vi "Pose_Estimation.vi"() -> ()   [LabVIEW 2019]
uses:
  Hardware/Drive/Drive_Hardware_Globals.vi
  <vilib>/Rock Robotics/WPI/ThirdParty/Phoenix-LabVIEW/Motor Controller/Get/CTRE_Phoenix_MotorController_GetSelectedSensorData.vi
  Globals/Sensor_Values.vi
panel:
  out "Y pos (in)":dbl
  out "X pos (in)":dbl
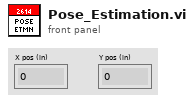
[diagram p1: front panel]
types:
  T1 = typedef "WPI_MotorControlDeviceRef.ctl" = cluster{"DeviceStatus":errorcluster, "Type":T2, "PWM":cluster{"PWM Channel":T3, "DeadBand":T4}, "CAN":cluster{"Device Number":u8, "SetOutput VI Ref":variant, "GetOutput VI Ref":variant, "Enable VI Ref":variant, "Disable VI Ref":variant, "Data":variant}, "Invert":bool, "DIO PWM":cluster{"PWM \"Enable\" Channel":T3, "DIOChannel":T5, "PWM Rate":dbl}}
  T2 = typedef "WPI_MotorControlType.ctl" = enum16{"PWM", "CAN", "DIO PWM"}
  T3 = typedef "FPGA_DIOPWMChannel.ctl" = enum8{"PWM 0", "PWM 1", "PWM 2", "PWM 3", "PWM 4", "PWM 5", "PWM 6", "PWM 7", "PWM 8", "PWM 9", "PWM MXP 0", "PWM MXP 1", "PWM MXP 2", "PWM MXP 3", "PWM MXP 4", "PWM MXP 5", "PWM MXP 6", "PWM MXP 7", "PWM MXP 8", "PWM MXP 9", "Invalid"}
  T4 = typedef "WPI_PWMDeadband.ctl" = cluster{"Name":string, "maxPositivePwm":i32, "minPositivePwm":i32, "centerPwm":i32, "maxNegativePwm":i32, "minNegativePwm":i32, "angularRange":u16}
  T5 = typedef "FPGA_DIOChannel.ctl" = enum8{"DIO 0", "DIO 1", "DIO 2", "DIO 3", "DIO 4", "DIO 5", "DIO 6", "DIO 7", "DIO 8", "DIO 9", "DIO MXP 0", "DIO MXP 1", "DIO MXP 2", "DIO MXP 3", "DIO MXP 4", "DIO MXP 5", "DIO MXP 6", "DIO MXP 7", "DIO MXP 8", "DIO MXP 9", "DIO MXP 10", "DIO MXP 11", "DIO MXP 12", "DIO MXP 13", "DIO MXP 14", "DIO MXP 15", "SPI Port CS1", "SPI Port CS2", "SPI Port CS3", "SPI Port MISO", "SPI Port MOSI", "Invalid"}
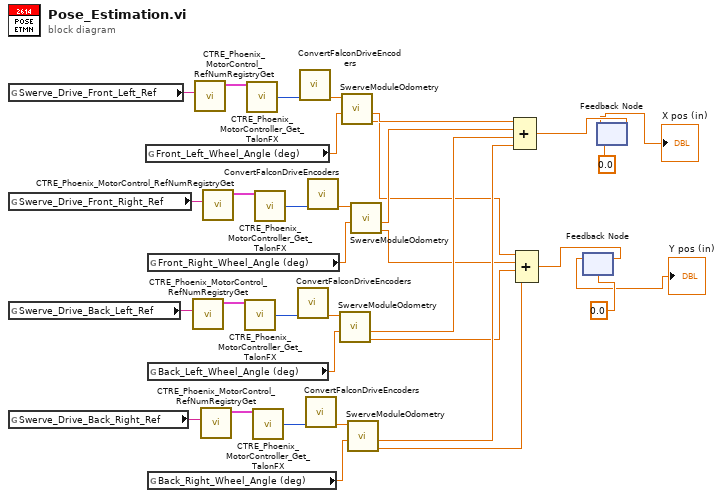
[diagram p0: block diagram]
diagram:
  n1 = global read "Drive_Hardware_Globals.vi" "Swerve_Drive_Front_Left_Ref"() -> (w33:string)
  n2 = global read "Drive_Hardware_Globals.vi" "Swerve_Drive_Front_Right_Ref"() -> (w32:string)
  n3 = global read "Drive_Hardware_Globals.vi" "Swerve_Drive_Back_Left_Ref"() -> (w34:string)
  n4 = global read "Drive_Hardware_Globals.vi" "Swerve_Drive_Back_Right_Ref"() -> (w31:string)
  n5 = global read "Sensor_Values.vi" "Front_Left_Wheel_Angle (deg)"() -> (w17:dbl)
  n6 = global read "Sensor_Values.vi" "Front_Right_Wheel_Angle (deg)"() -> (w18:dbl)
  n7 = global read "Sensor_Values.vi" "Back_Left_Wheel_Angle (deg)"() -> (w15:dbl)
  n8 = global read "Sensor_Values.vi" "Back_Right_Wheel_Angle (deg)"() -> (w16:dbl)
  n9 = call <vilib>:"CTRE_Phoenix_MotorControl_RefNumRegistryGet.vi"("refnum name"=w34) -> ("PhoenixMotorControlDevRef"=w28:T1)  [unwired: 9 in, 1 out]
  n10 = call <vilib>:"CTRE_Phoenix_MotorControl_RefNumRegistryGet.vi"("refnum name"=w33) -> ("PhoenixMotorControlDevRef"=w30:T1)  [unwired: 9 in, 1 out]
  n11 = call <vilib>:"CTRE_Phoenix_MotorControl_RefNumRegistryGet.vi"("refnum name"=w31) -> ("PhoenixMotorControlDevRef"=w27:T1)  [unwired: 9 in, 1 out]
  n12 = call <vilib>:"CTRE_Phoenix_MotorControl_RefNumRegistryGet.vi"("refnum name"=w32) -> ("PhoenixMotorControlDevRef"=w29:T1)  [unwired: 9 in, 1 out]
  n13 = call-poly <vilib>:"CTRE_Phoenix_MotorController_Get_TalonFX.vi"("PhoenixMotorControlDevRef"=w28) -> ("Velocity (Raw Sensor Units per 100 ms)"=w24:i32)  [unwired: 11 in, 3 out]
  n14 = call-poly <vilib>:"CTRE_Phoenix_MotorController_Get_TalonFX.vi"("PhoenixMotorControlDevRef"=w30) -> ("Velocity (Raw Sensor Units per 100 ms)"=w26:i32)  [unwired: 11 in, 3 out]
  n15 = call-poly <vilib>:"CTRE_Phoenix_MotorController_Get_TalonFX.vi"("PhoenixMotorControlDevRef"=w27) -> ("Velocity (Raw Sensor Units per 100 ms)"=w23:i32)  [unwired: 11 in, 3 out]
  n16 = call-poly <vilib>:"CTRE_Phoenix_MotorController_Get_TalonFX.vi"("PhoenixMotorControlDevRef"=w29) -> ("Velocity (Raw Sensor Units per 100 ms)"=w25:i32)  [unwired: 11 in, 3 out]
  n17 = call "ConvertFalconDriveEncoders.vi"("Velocity (Raw Sensor Units per 100 ms)"=w24) -> ("Velocity (ft/s)"=w20:dbl)  [unwired: 14 in]
  n18 = call "ConvertFalconDriveEncoders.vi"("Velocity (Raw Sensor Units per 100 ms)"=w26) -> ("Velocity (ft/s)"=w22:dbl)  [unwired: 14 in]
  n19 = call "ConvertFalconDriveEncoders.vi"("Velocity (Raw Sensor Units per 100 ms)"=w23) -> ("Velocity (ft/s)"=w19:dbl)  [unwired: 14 in]
  n20 = call "ConvertFalconDriveEncoders.vi"("Velocity (Raw Sensor Units per 100 ms)"=w25) -> ("Velocity (ft/s)"=w21:dbl)  [unwired: 14 in]
  n21 = call "SwerveModuleOdometry.vi"("Wheel Azimuth (deg)"=w15, "Velocity (ft/s)"=w20) -> ("Delta Y (in)"=w8:dbl, "Delta X (in)"=w12:dbl)  [unwired: 4 in, 2 out]
  n22 = call "SwerveModuleOdometry.vi"("Wheel Azimuth (deg)"=w17, "Velocity (ft/s)"=w22) -> ("Delta Y (in)"=w10:dbl, "Delta X (in)"=w14:dbl)  [unwired: 4 in, 2 out]
  n23 = call "SwerveModuleOdometry.vi"("Wheel Azimuth (deg)"=w16, "Velocity (ft/s)"=w19) -> ("Delta Y (in)"=w7:dbl, "Delta X (in)"=w11:dbl)  [unwired: 4 in, 2 out]
  n24 = call "SwerveModuleOdometry.vi"("Wheel Azimuth (deg)"=w18, "Velocity (ft/s)"=w21) -> ("Delta Y (in)"=w9:dbl, "Delta X (in)"=w13:dbl)  [unwired: 4 in, 2 out]
  n25 = Compound Arithmetic op=ADD(w14, w13, w12, w11) -> (w5:dbl)
  n26 = Compound Arithmetic op=ADD(w10, w9, w8, w7) -> (w2:dbl)
  n27 = feedback #1(0.0) -> (→"Y pos (in)":dbl)
  n28 = feedback-in #1(w2) -> ()
  n29 = feedback-in #2(w5) -> ()
  n30 = feedback #2(0.0) -> (→"X pos (in)":dbl)
